vi "Load Config.vi"(6 "Constants":refnum<class "Sequence Constants.lvclass">, 8 "error in (no error)":refnum<class "MultiErrors.lvclass">, 10 "Config Element":refnum<class "Config Element.lvclass">, 11 "Transition Config in":refnum<class "Transition Config.lvclass">) -> (0 "error out":refnum<class "MultiErrors.lvclass">, 3 "Transition Config out":refnum<class "Transition Config.lvclass">)   [LabVIEW 2020, in "VolatusSeqConfig.lvlib" / "Transition Config.lvclass"]
uses:
  Transition Config.lvclass
  VolatusErrorUtilities/MultiErrors/MultiErrors.lvclass
  lv-cdm/CDM-Config/Config Element/Config Element.lvclass
  Condition Logic.ctl
  Transition Config.lvclass/Transition Config.ctl
  VolatusSeqConfig.lvlib
  VolatusErrorUtilities/VolatusErrorUtilities.lvlib
  Sequence Constants/Sequence Constants.lvclass
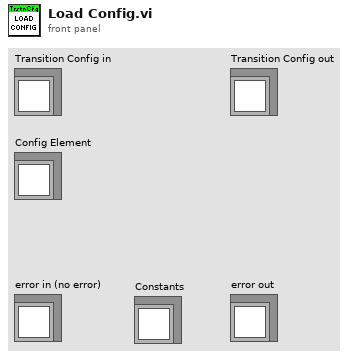
[diagram p1: front panel]
types:
  T1 = typedef "VolatusSeqConfig.lvlib/Condition Logic.ctl" = enum16{"All", "Any"}
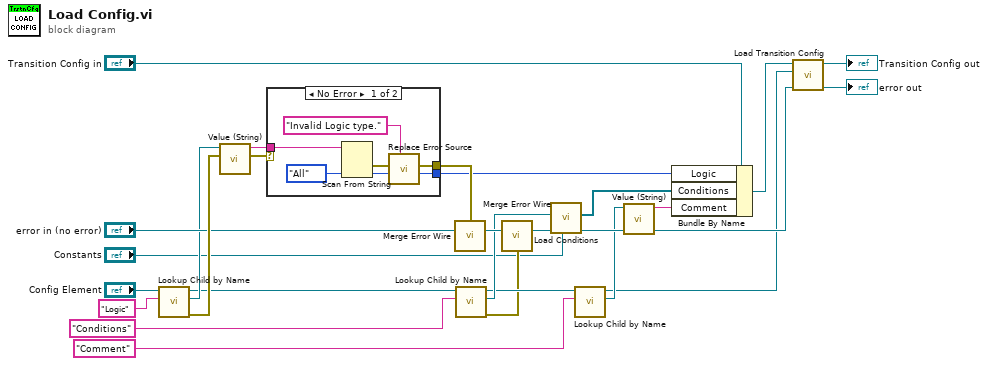
[diagram p0: block diagram]
diagram:
  n1 = call "Lookup Child by Name.vi"("Name"="Logic", "Config Element in"="Config Element") -> ("error out"=w26:errorcluster, "Child"=w17:refnum<class "Config Element.lvclass">, "Config Element out"=w13:refnum<class "Config Element.lvclass">)  [unwired: 6 in, 1 out]
  n2 = call "Value (String).vi"("error in (no error)"=w26, "Config Element in"=w17) -> ("error out"=w4:errorcluster, "String Value"=w16:string)  [unwired: 8 in]
  n3 = case shown="No Error" w4 {
    selector: w4 -> [_ w34]
    tunnel: w16 -> [w33 _]
    tunnel: [w32 _] -> w14
    tunnel: [w30 w34] -> w27
    frame No Error {
      n4 = Scan From String(input string=w33, default 1=Condition_Logic."All" ("Condition Logic")) -> (error out=w31:errorcluster, output 1=w32:T1)  [unwired: 3 in, 2 out]
      n5 = call "Replace Error Source.vi"("New Source"="Invalid Logic type." ("Prepend String"), "error in (no error)"=w31) -> ("error out"=w30:errorcluster)  [unwired: 9 in]
    }
    frame Error {
    }
  }
  n6 = call "Merge Error Wire.vi"("error in (no error)"=w27, "MultiErrors in"="error in (no error)") -> ("MultiErrors out"=w24:refnum<class "MultiErrors.lvclass">)  [unwired: 13 in]
  n7 = call "Lookup Child by Name.vi"("Name"="Conditions", "Config Element in"=w13) -> ("error out"=w3:errorcluster, "Child"=w11:refnum<class "Config Element.lvclass">, "Config Element out"=w8:refnum<class "Config Element.lvclass">)  [unwired: 6 in, 1 out]
  n8 = call "Merge Error Wire.vi"("error in (no error)"=w3, "MultiErrors in"=w24) -> ("MultiErrors out"=w2:refnum<class "MultiErrors.lvclass">)  [unwired: 13 in]
  n9 = call "Load Conditions.vi"("Constants"="Constants", "error in (no error)"=w2, "Config Element"=w11) -> ("error out"=w25:refnum<class "MultiErrors.lvclass">, "Conditions"=w10:refnum<class "Condition Config.lvclass">[])  [unwired: 7 in]
  n10 = call "Lookup Child by Name.vi"("Name"="Comment", "Config Element in"=w8) -> ("Child"=w7:refnum<class "Config Element.lvclass">, "Config Element out"=w5:refnum<class "Config Element.lvclass">)  [unwired: 6 in, 2 out]
  n11 = call "Value (String).vi"("Config Element in"=w7) -> ("String Value"=w6:string)  [unwired: 9 in, 1 out]
  n12 = Bundle By Name(cluster="Transition Config in", "Logic"=w14, "Conditions"=w10, "Comment"=w6) -> (w15:refnum<class "Transition Config.lvclass">)
  n13 = call-dynamic "Load Transition Config.vi"("error in (no error)"=w25, "Config Element"=w5, "Transition Config in"=w15) -> ("error out"=→"error out":refnum<class "MultiErrors.lvclass">, "Transition Config out"=→"Transition Config out":refnum<class "Transition Config.lvclass">)  [unwired: 7 in]
